vi "receive-waveArray.vi"(6 "波形数组in":dbl[](array[numeric]), 8 "VCI_CAN_OBJ":T2, 10 "输出数组":T1(array[cluster])) -> (2 "波形数组out":dbl[](array[numeric]))   [LabVIEW 2016]
panel:
  out "添加的数组":u64[](array[numeric])
  out "result":u64
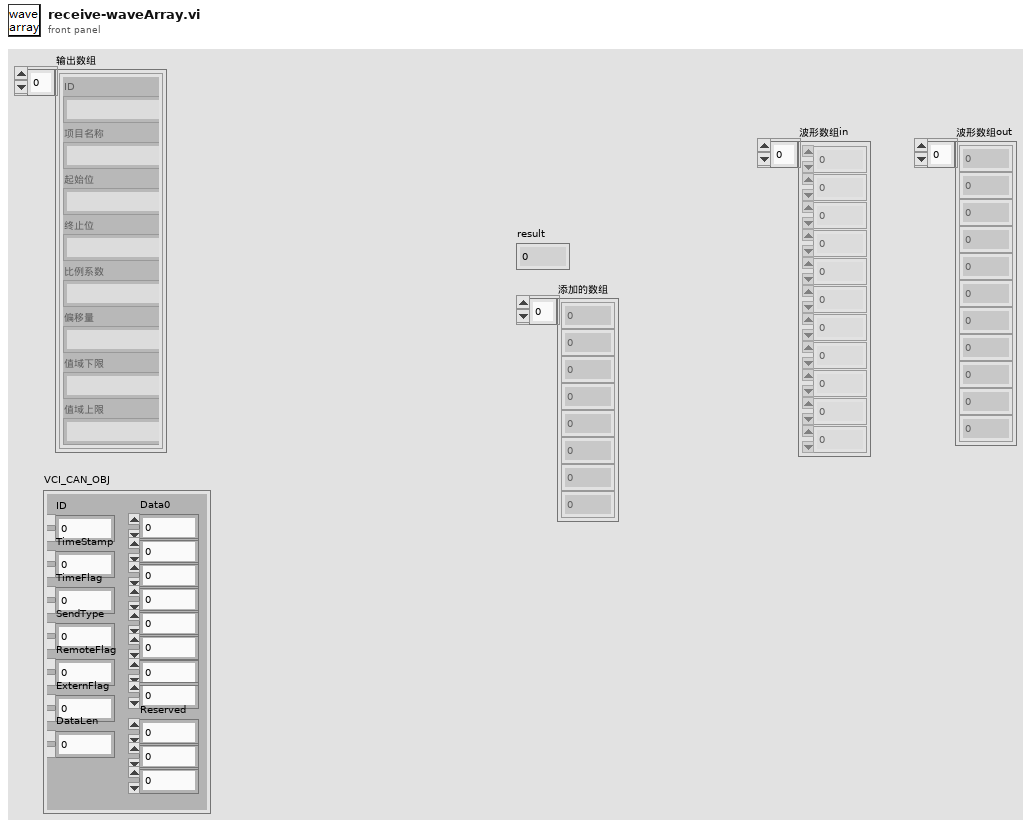
[diagram p1: front panel]
types:
  T1 = cluster{"ID":string, "项目名称":string, "起始位":string, "终止位":string, "比例系数":string, "偏移量":string, "值域下限":string, "值域上限":string}[]
  T2 = cluster{"ID":u32, "TimeStamp":u32, "TimeFlag":u8, "SendType":i8, "RemoteFlag":u8, "ExternFlag":u8, "DataLen":u8, "Data0":u64, "Data1":u64, "Data2":u64, "Data3":u64, "Data4":u64, "Data5":u64, "Data6":u64, "Data7":u64, "Reserved":u8, u8, u8}
  T3 = cluster{"ID":u32, "起始位":u8, "终止位":u8, "比例系数":dbl, "偏移量":dbl}[]
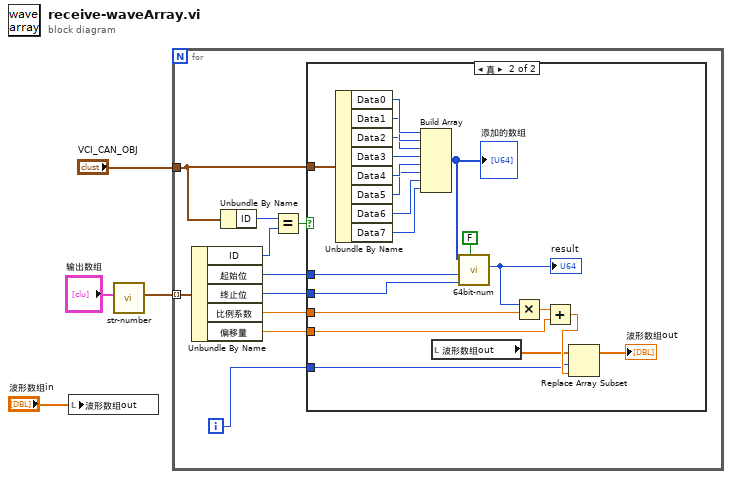
[diagram p0: block diagram]
diagram:
  n1 = local write "波形数组out"("波形数组in") -> ()
  n2 = call "str-number.vi"("输出数组"="输出数组") -> ("数组"=w2:T3)  [unwired: 10 in]
  n3 = for {
    tunnel: w2 -> [w14] mode=indexing
    tunnel: "VCI_CAN_OBJ" -> [w10]
    i -> [w5]
    n4 = Unbundle By Name(w14) -> ("ID"=w7:u32, "起始位"=w13:u8, "终止位"=w12:u8, "比例系数"=w9:dbl, "偏移量"=w8:dbl)
    n5 = Unbundle By Name(w10) -> ("ID"=w6:u32)
    n6 = Equal?(x=w6, y=w7) -> (x = y?=w11:bool)
    n7 = case shown="真" w11 {
      tunnel: w13 -> [_ w35]
      tunnel: w12 -> [_ w34]
      tunnel: w10 -> [_ w25]
      tunnel: w9 -> [_ w22]
      tunnel: w8 -> [_ w19]
      tunnel: w5 -> [_ w17]
      frame False {
      }
      frame True {
        n8 = Unbundle By Name(w25) -> ("Data0"=w33:u64, "Data1"=w32:u64, "Data2"=w31:u64, "Data3"=w30:u64, "Data4"=w29:u64, "Data5"=w28:u64, "Data6"=w27:u64, "Data7"=w26:u64)
        n9 = Build Array(w33, w32, w31, w30, w29, w28, w27, w26) -> (w24:u64[])
        "添加的数组" <- w24
        n10 = local read "波形数组out"() -> (w15:dbl[])
        n11 = call "64bit-num.vi"("format"=FALSE, "end bit"=w34, "start bit"=w35, "framedata"=w24) -> ("result"=w21:u64)  [unwired: 7 in]
        "result" <- w21
        n12 = Multiply(x=w21, y=w22) -> (x*y=w20:dbl)
        n13 = Add(x=w20, y=w19) -> (x+y=w18:dbl)
        n14 = Replace Array Subset(array=w15, new element=w18, index=w17) -> (→"波形数组out":dbl[])
      }
    }
  }
